vi "New position calculator.vi"() -> ()   [LabVIEW 2015]
panel:
  out "dY":dbl
  out "dX":dbl
  in  "Initial angle (radians)":dbl
  in  "Robot Width":dbl
  in  "Encoder Position Right Old":dbl
  in  "Encoder Position Left Old":dbl
  in  "Encoder Position Right New":dbl
  in  "Encoder Position Left New":dbl
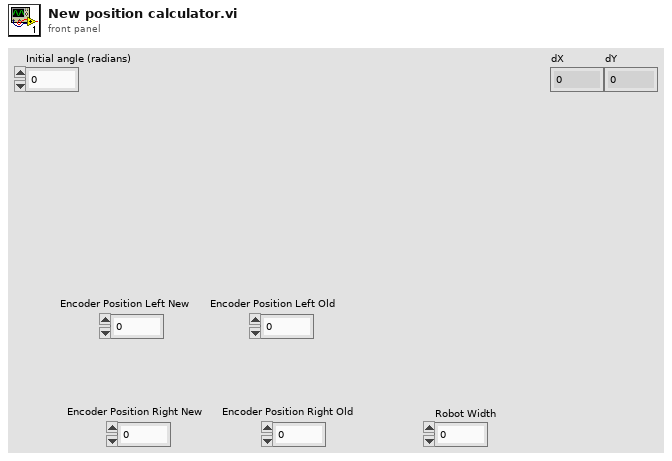
[diagram p1: front panel]
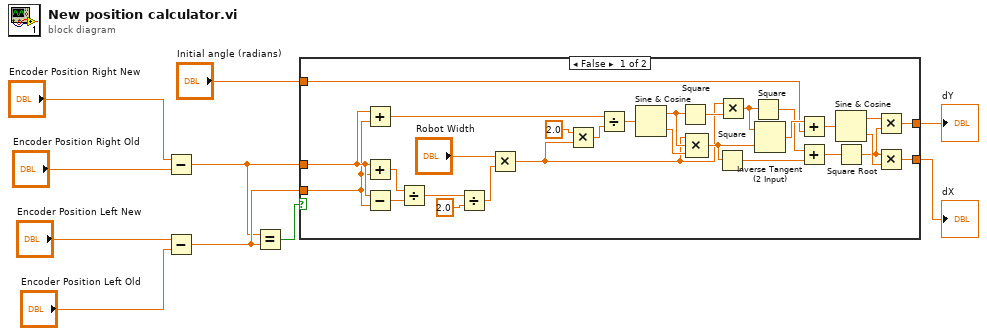
[diagram p0: block diagram]
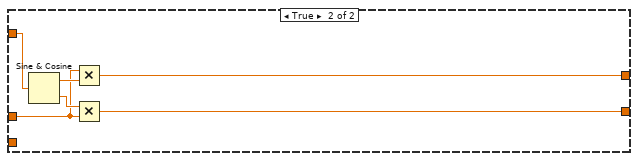
[diagram p2: hidden frame]
diagram:
  n1 = Subtract(x="Encoder Position Right New", y="Encoder Position Right Old") -> (x-y=w4:dbl)
  n2 = Subtract(x="Encoder Position Left New", y="Encoder Position Left Old") -> (x-y=w5:dbl)
  n3 = Equal?(x=w4, y=w5) -> (x = y?=w3:bool)
  n4 = case shown="False" w3 {
    tunnel: "Initial angle (radians)" -> [w30 w45]
    tunnel: [w25 w43] -> w2
    tunnel: [w27 w40] -> w1
    tunnel: w5 -> [w19 _]
    tunnel: w4 -> [w20 w41]
    frame False {
      n5 = Add(x=w20, y=w19) -> (x+y=w36:dbl)
      n6 = Add(x=w20, y=w19) -> (x+y=w39:dbl)
      n7 = Subtract(x=w20, y=w19) -> (x-y=w38:dbl)
      n8 = Divide(x=w39, y=w38) -> (x/y=w35:dbl)
      n9 = Divide(x=w35, y=2.0) -> (x/y=w34:dbl)
      n10 = Multiply(x="Robot Width", y=w34) -> (x*y=w12:dbl)
      n11 = Multiply(x=2.0, y=w12) -> (x*y=w37:dbl)
      n12 = Divide(x=w36, y=w37) -> (x/y=w18:dbl)
      n13 = Sine & Cosine(0:w18) -> (1:w14:dbl, 2:w16:dbl)
      n14 = Square(x=w14) -> (x^2=w13:dbl)
      n15 = Compound Arithmetic op=MULTIPLY(w12, w14, w16) -> (w15:dbl)
      n16 = Square(x=w15) -> (x^2=w22:dbl)
      n17 = Multiply(x=w12, y=w13) -> (x*y=w11:dbl)
      n18 = Square(x=w11) -> (x^2=w23:dbl)
      n19 = Inverse Tangent (2 Input)(1:w15, 2:w11) -> (0:w31:dbl)
      n20 = Add(x=w31, y=w30) -> (x+y=w29:dbl)
      n21 = Add(x=w23, y=w22) -> (x+y=w24:dbl)
      n22 = Sine & Cosine(0:w29) -> (1:w28:dbl, 2:w26:dbl)
      n23 = Square Root(x=w24) -> (sqrt(x)=w21:dbl)
      n24 = Multiply(x=w28, y=w21) -> (x*y=w27:dbl)
      n25 = Multiply(x=w21, y=w26) -> (x*y=w25:dbl)
    }
    frame True {
      n26 = Sine & Cosine(0:w45) -> (1:w42:dbl, 2:w44:dbl)
      n27 = Multiply(x=w41, y=w42) -> (x*y=w40:dbl)
      n28 = Multiply(x=w44, y=w41) -> (x*y=w43:dbl)
    }
  }
  "dX" <- w2
  "dY" <- w1
